vi "fileRedGreenRegistrationLoad.vi"(0 "redGreenRegistrationFilePath":string) -> (4 "denormParam":dbl[](array[numeric]), 5 "ctrl":dbl[][](array[numeric]), 6 "param":dbl[](array[numeric]), 7 "red (model)":dbl[][](array[numeric]), 8 "normParam":dbl[](array[numeric]), 9 "green (scene)":dbl[][](array[numeric]))   [LabVIEW 2017]
uses:
  <vilib>/Utility/file.llb/Read Delimited Spreadsheet (DBL).vi
  globalUtilities.vi
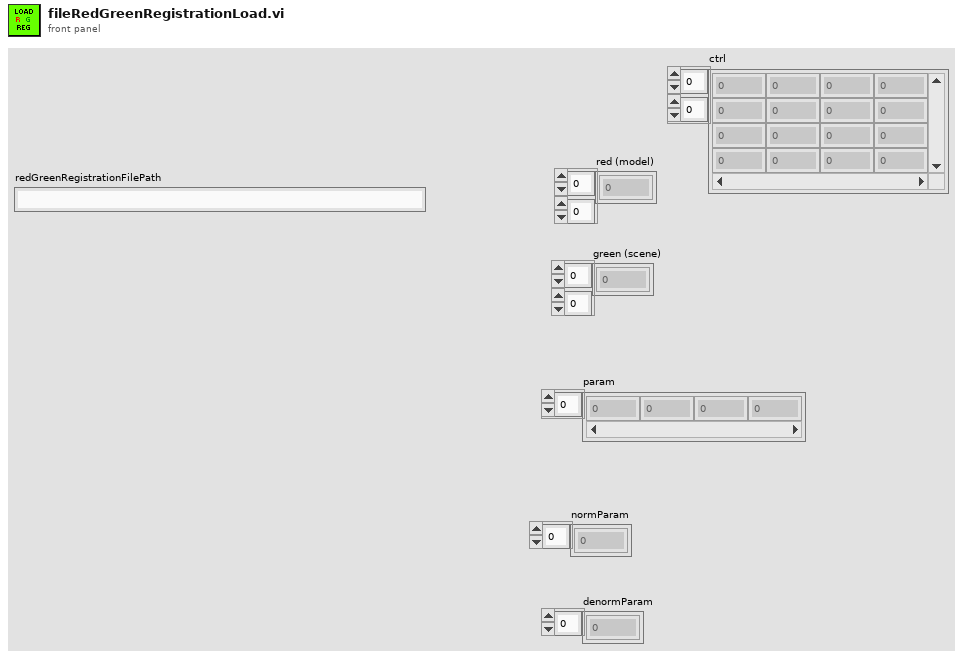
[diagram p1: front panel]
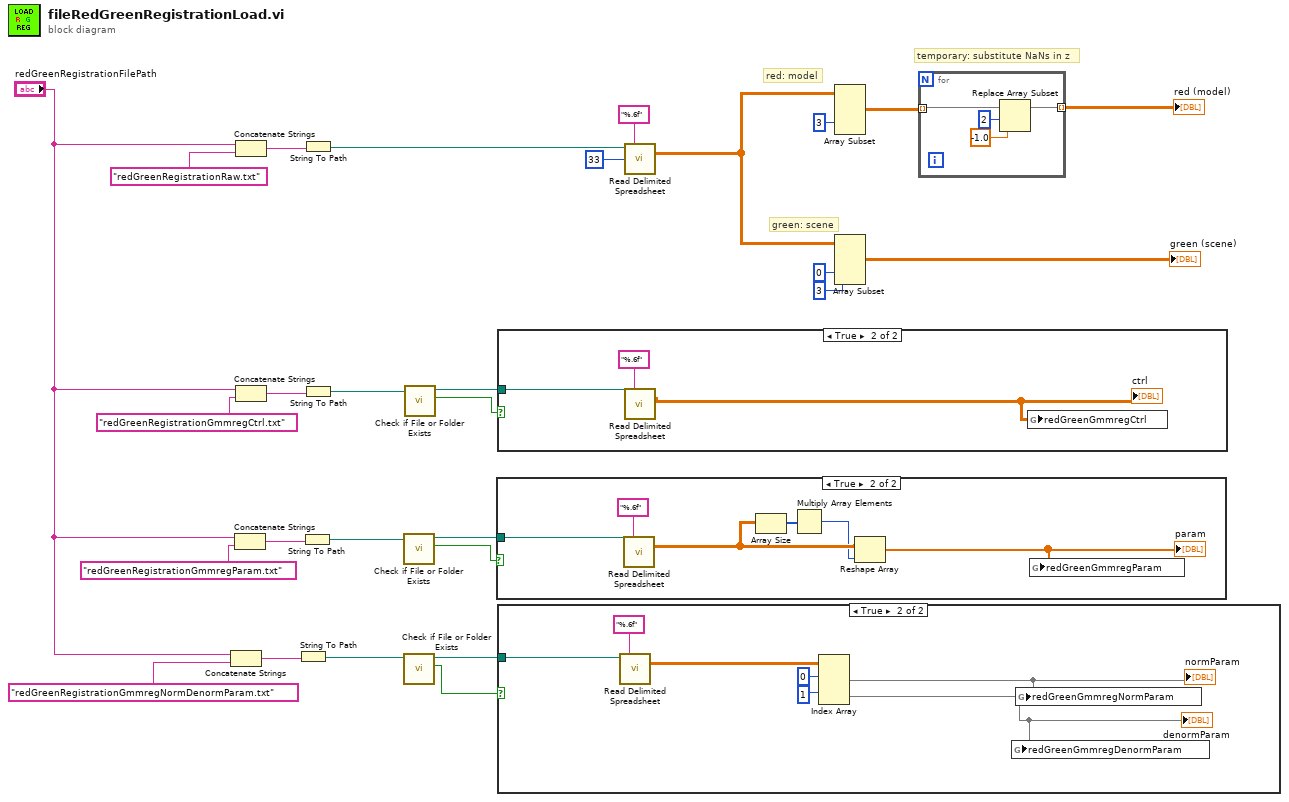
[diagram p0: block diagram]
diagram:
  # "temporary: substitute NaNs in z"
  # "red: model"
  # "green: scene"
  n1 = Concatenate Strings("redGreenRegistrationFilePath", "redGreenRegistrationGmmregNormDenormParam.txt" ("string")) -> (w15:string)
  n2 = Concatenate Strings("redGreenRegistrationFilePath", "redGreenRegistrationGmmregParam.txt" ("string")) -> (w17:string)
  n3 = Concatenate Strings("redGreenRegistrationFilePath", "redGreenRegistrationRaw.txt" ("string")) -> (w18:string)
  n4 = Concatenate Strings("redGreenRegistrationFilePath", "redGreenRegistrationGmmregCtrl.txt" ("string")) -> (w2:string)
  n5 = String To Path(string=w15) -> (path=w12:path)
  n6 = String To Path(string=w17) -> (path=w13:path)
  n7 = String To Path(string=w18) -> (path=w20:path)
  n8 = String To Path(string=w2) -> (path=w4:path)
  n9 = call <vilib>:"Check if File or Folder Exists.vi"("path"=w13) -> ("file or folder exists?"=w9:bool, "dup path"=w11:path)  [unwired: 8 in, 1 out]
  n10 = call <vilib>:"Check if File or Folder Exists.vi"("path"=w12) -> ("file or folder exists?"=w8:bool, "dup path"=w10:path)  [unwired: 8 in, 1 out]
  n11 = call <vilib>:"Check if File or Folder Exists.vi"("path"=w4) -> ("file or folder exists?"=w6:bool, "dup path"=w5:path)  [unwired: 8 in, 1 out]
  n12 = case shown="True" w9 {
    tunnel: w11 -> [_ w33]
    frame False {
    }
    frame True {
      n13 = call-poly <vilib>:"Read Delimited Spreadsheet.vi"("file path (dialog if empty)"=w33, "format (%.3f)"="%.6f") -> ("all rows"=w31:dbl[][])  [unwired: 8 in, 5 out]
      n14 = Array Size(array=w31) -> (size(s)=w32:i32[])
      n15 = Multiply Array Elements(1:w32) -> (0:w30:i32)
      n16 = Reshape Array(w31, w30) -> (w29:dbl[])
      "param" <- w29
      n17 = global write "globalUtilities.vi" "redGreenGmmregParam"(w29) -> ()
    }
  }
  n18 = case shown="True" w6 {
    tunnel: w5 -> [_ w36]
    frame False {
    }
    frame True {
      n19 = call-poly <vilib>:"Read Delimited Spreadsheet.vi"("file path (dialog if empty)"=w36, "format (%.3f)"="%.6f") -> ("all rows"=w35:dbl[][])  [unwired: 8 in, 5 out]
      "ctrl" <- w35
      n20 = global write "globalUtilities.vi" "redGreenGmmregCtrl"(w35) -> ()
    }
  }
  n21 = case shown="True" w8 {
    tunnel: w10 -> [_ w40]
    frame False {
    }
    frame True {
      n22 = call-poly <vilib>:"Read Delimited Spreadsheet.vi"("file path (dialog if empty)"=w40, "format (%.3f)"="%.6f") -> ("all rows"=w43:dbl[][])  [unwired: 8 in, 5 out]
      n23 = Index Array(array=w43, index (row) #1=0 ("index (row)"), index (row) #2=1 ("disabled index (col)")) -> (element #1=w39:dbl[], element #2=w38:dbl[])  [unwired: 2 in]
      "normParam" <- w39
      "denormParam" <- w38
      n24 = global write "globalUtilities.vi" "redGreenGmmregDenormParam"(w38) -> ()
      n25 = global write "globalUtilities.vi" "redGreenGmmregNormParam"(w39) -> ()
    }
  }
  n26 = call-poly <vilib>:"Read Delimited Spreadsheet.vi"("file path (dialog if empty)"=w20, "format (%.3f)"="%.6f", "start of read offset (chars.:0)"=33) -> ("all rows"=w23:dbl[][])  [unwired: 7 in, 5 out]
  n27 = Array Subset(array=w23, index (col)=3 ("index")) -> (w22:dbl[][])  [unwired: 3 in]
  n28 = Array Subset(array=w23, index (col)=0 ("index"), length (col)=3 ("length")) -> (→"green (scene)":dbl[][])  [unwired: 2 in]
  n29 = for {
    tunnel: w22 -> [w48] mode=indexing
    tunnel: [w45] -> w7 mode=indexing
    n30 = Replace Array Subset(array=w48, new element=-1.0 ("new element/subarray"), index=2) -> (w45:dbl[])
  }
  "red (model)" <- w7
